vi "SetSignalParams.vi"(8 "error in (no error)":errorcluster, 10 "Variant":variant, 11 "PmuTestFunctions in":refnum<class "PmuTestFunctions.lvclass">) -> (0 "error out":errorcluster, 3 "PmuTestFunctions out":refnum<class "PmuTestFunctions.lvclass">)   [LabVIEW 2018, in "Functions.lvlib" / "PmuTestFunctions.lvclass"]
uses:
  PmuTestFunctions.lvclass
  PmuTestFunctions.lvclass/PmuTestFunctions.ctl
  Accessors/Write PmuTestParams.vi
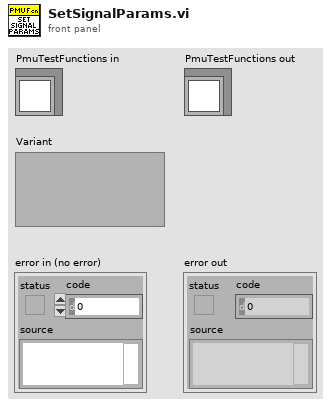
[diagram p1: front panel]
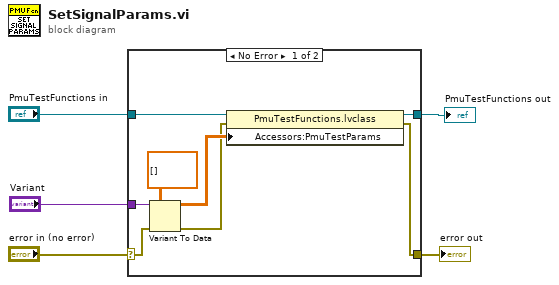
[diagram p0: block diagram]
diagram:
  n1 = case shown="No Error" "error in (no error)" {
    selector: "error in (no error)" -> [w11 w15]
    tunnel: "PmuTestFunctions in" -> [w10 w14]
    tunnel: "Variant" -> [w13 _]
    tunnel: [w6 w15] -> w2
    tunnel: [w9 w14] -> w1
    frame No Error {
      n2 = Variant To Data(error in=w11, type=dbl[][] [], Variant=w13) -> (data=w8:dbl[][], error out=w7:errorcluster)
      n3 = property class="PmuTestFunctions.lvclass"(reference=w10, error in=w7, "Accessors:PmuTestParams"=w8) -> (reference out=w9:refnum<class "PmuTestFunctions.lvclass">, error out=w6:errorcluster)
    }
    frame Error {
    }
  }
  "error out" <- w2
  "PmuTestFunctions out" <- w1
